vi "New Data File.vi"(6 "Plot type":T1, 8 "error in (no error)":errorcluster, 9 "New plot if not open":bool, 10 "File":path, 11 "Application Controller in":refnum<class "Application Controller.lvclass">) -> (0 "error out":errorcluster, 3 "Application Controller out":refnum<class "Application Controller.lvclass">)   [LabVIEW 2016, in "Application Controller.lvclass"]
uses:
  Application Controller.lvclass
  Plots/Plot types.ctl
  Application Controller.lvclass/Application Controller.ctl
  Plots/Plot Messages/Add file Msg/Add file Msg.lvclass/Add file Msg.ctl
  <vilib>/ActorFramework/Message Enqueuer/Message Enqueuer.lvclass/Message Enqueuer.ctl
  <vilib>/ActorFramework/Message Enqueuer/Enqueue.vi
  Plots/Plot Messages/Add file Msg/Add file Msg.lvclass
  C:/Program Files/National Instruments/LabVIEW 2016/vi.lib/ActorFramework/Message/Message.lvclass
  <vilib>/ActorFramework/Message Priority Queue/Priority Enqueue.vi
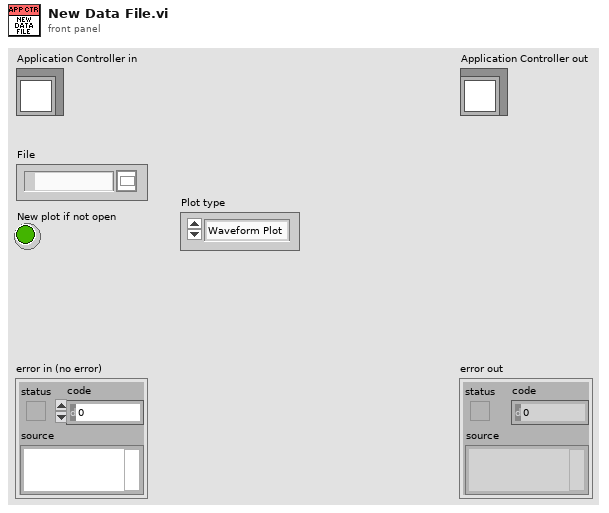
[diagram p1: front panel]
types:
  T1 = typedef "Plot types.ctl" = enum16{"Waveform Plot", "XY Plot", "Full XY"}
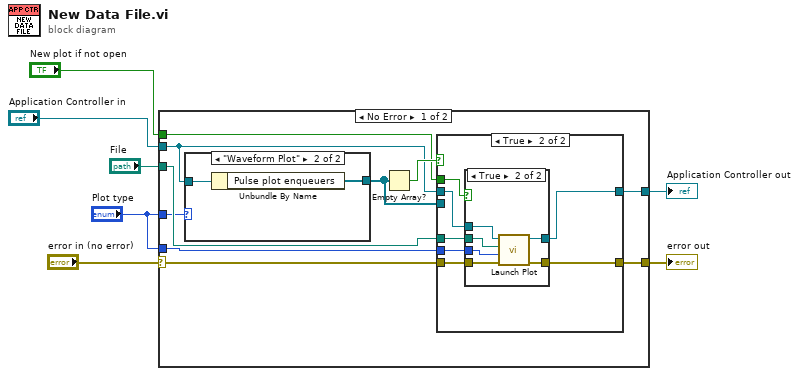
[diagram p0: block diagram]
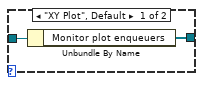
[diagram p2: hidden frame]
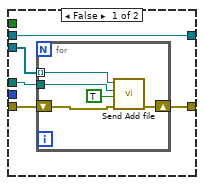
[diagram p3: hidden frame]
diagram:
  n1 = case shown="No Error" "error in (no error)" {
    selector: "error in (no error)" -> [w12 w48]
    tunnel: [w11 w48] -> w3
    tunnel: [w13 w47] -> w2
    tunnel: "Application Controller in" -> [w14 w47]
    tunnel: "File" -> [w15 _]
    tunnel: "New plot if not open" -> [w10 _]
    tunnel: "Plot type" -> [w9 _]
    tunnel: "Plot type" -> [w8 _]
    frame No Error {
      n2 = case shown="\"Waveform Plot\"" w8 {
        tunnel: [w19 w21] -> w17
        tunnel: w14 -> [w18 w20]
        frame "XY Plot", Default {
          n3 = Unbundle By Name(w18) -> ("Monitor plot enqueuers"=w19:refnum<class "Message Enqueuer.lvclass">[])
        }
        frame "Waveform Plot" {
          n4 = Unbundle By Name(w20) -> ("Pulse plot enqueuers"=w21:refnum<class "Message Enqueuer.lvclass">[])
        }
      }
      n5 = Empty Array?(array=w17) -> (empty?=w16:bool)
      n6 = case shown="True" w16 {
        tunnel: w12 -> [w25 w38]
        tunnel: [w24 w37] -> w11
        tunnel: w14 -> [w23 w36]
        tunnel: [w23 w35] -> w13
        tunnel: w15 -> [w22 w34]
        tunnel: w17 -> [w26 _]
        tunnel: w10 -> [_ w33]
        tunnel: w9 -> [_ w32]
        frame False {
          n7 = for {
            tunnel: w26 -> [w31] mode=indexing
            tunnel: w22 -> [w30]
            shift-right: [w28] -> w24
            shift-left: w25 -> [w29]
            n8 = call "Send Add file.vi"("error in (no error)"=w29, "Insert in front"=TRUE, "File Path Control"=w30, "Message Enqueuer"=w31) -> ("error out"=w28:errorcluster)  [unwired: 6 in, 1 out]
          }
        }
        frame True {
          n9 = case shown="True" w33 {
            tunnel: w38 -> [w40 w46]
            tunnel: [w40 w45] -> w37
            tunnel: w36 -> [w39 w44]
            tunnel: [w39 w43] -> w35
            tunnel: w34 -> [_ w42]
            tunnel: w32 -> [_ w41]
            frame False {
            }
            frame True {
              n10 = call-dynamic "Launch Plot.vi"("error in (no error)"=w46, "Plot type"=w41, "File Path Control"=w42, "Application Controller in"=w44) -> ("error out"=w45:errorcluster, "Application Controller out"=w43:refnum<class "Application Controller.lvclass">)  [unwired: 5 in, 1 out]
            }
          }
        }
      }
    }
    frame Error {
    }
  }
  "error out" <- w3
  "Application Controller out" <- w2
